vi "ECA200.vi"() -> ()   [LabVIEW 2020]
uses:
  <vilib>/Utility/miscctls.llb/LVComboBoxStrsAndValuesArrayTypeDef.ctl
panel:
  out "写入缓冲区":string
  in  "询问模式":bool
  out "返回数":u32
  out "读取缓冲区":string
  in  "测量":bool
  in  "确定按钮":bool
  in  "值":string(combo)
  in  "测量项":string(combo)
  in  "设置项":string(combo)
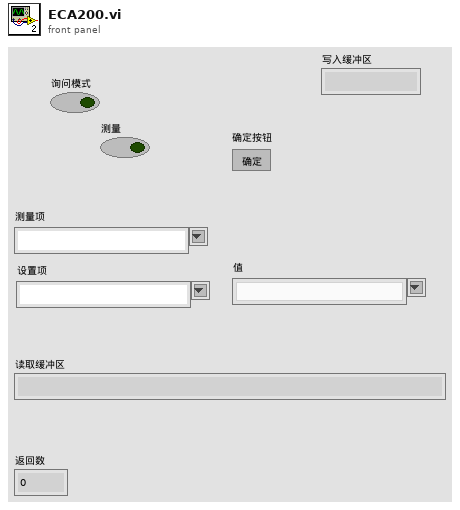
[diagram p1: front panel]
types:
  T1 = typedef "LVComboBoxStrsAndValuesArrayTypeDef.ctl" = cluster{"String":string, "Value":string}[]
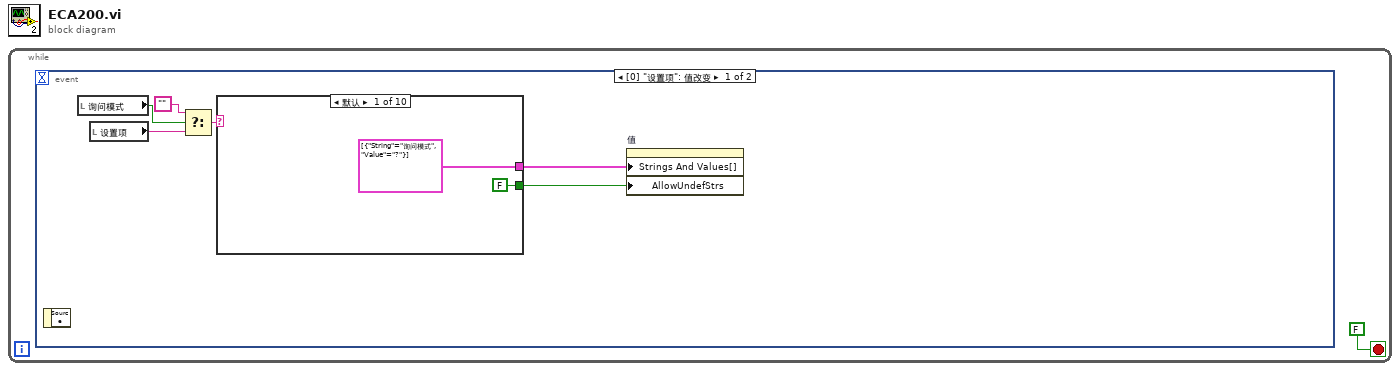
[diagram p0: block diagram]
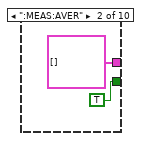
[diagram p2: hidden frame]
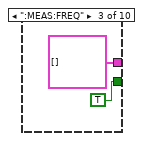
[diagram p3: hidden frame]
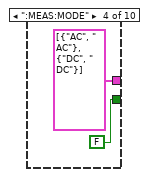
[diagram p4: hidden frame]
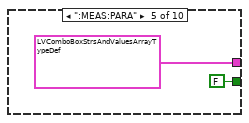
[diagram p5: hidden frame]
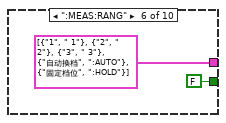
[diagram p6: hidden frame]
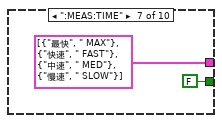
[diagram p7: hidden frame]
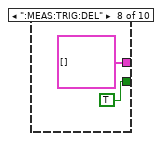
[diagram p8: hidden frame]
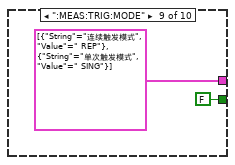
[diagram p9: hidden frame]
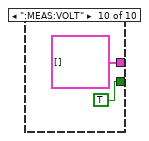
[diagram p10: hidden frame]
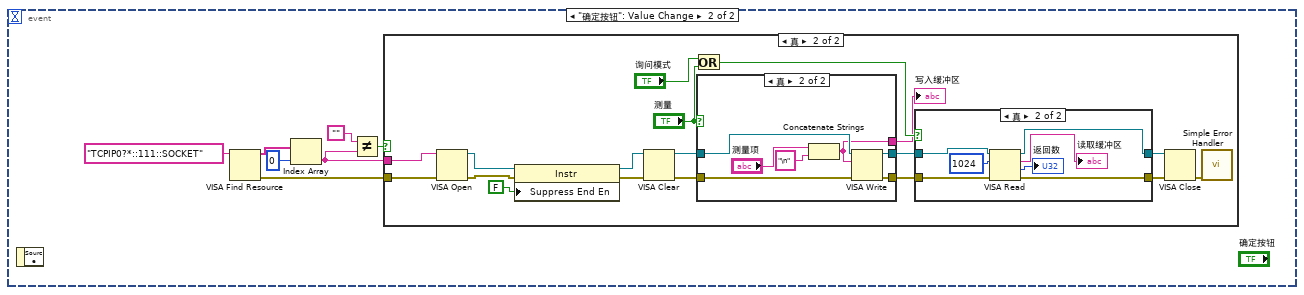
[diagram p11: hidden frame]
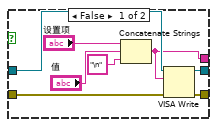
[diagram p14: hidden frame]
diagram:
  n1 = while {
    stop <- FALSE stop-if-true
    n2 = event shown="[0] \"设置项\": 值改变" {
      selector: _ -> [_ _]
      dyn-events: _ -> [_ _]
      timeout: _ -> [_ _]
      event "设置项": Value Change {
        n3 = event-data() -> ()  [unwired: 1 in, 1 out]
        n4 = local read "询问模式"() -> (w2:bool)
        n5 = local read "设置项"() -> (w5:string)
        n6 = Select(t="", s=w2, f=w5) -> (s? t:f=w7:string)
        n7 = case shown="默认" w7 {
          tunnel: [T1 [{"String"="询问模式", "Value"="?"}] ("字符串与值[]") T1 [] ("字符串与值[]") T1 [] ("字符串与值[]") T1 [{"String"="AC", "Value"=" AC"}, {"String"="DC", "Value"=" DC"}] ("字符串与值[]") T1 [{"String"="串联电感(Ls)", "Value"=" LS"}, {"String"="并联电感(Lp)", "Value"=" LP"}, {"String"="串联电容(Cs)", "Value"=" CS"}, {"String"="并联电容(Cp)", "Value"=" CP"}, {"String"="串联电阻(Rs)", "Value"=" RS"}, {"String"="并联电阻(Rp)", "Value"=" RP"}, {"String"="电抗(X)", "Value"=" X"}, {"String"="电纳(B)", "Value"=" B"}, {"String"="阻抗(Z)", "Value"=" Z"}, {"String"="导纳(Y)", "Value"=" Y"}, {"String"="损耗因数(D)", "Value"=" D"}, {"String"="品质因数(Q)", "Value"=" Q"}, {"String"="相位角(θ)", "Value"=" DEG"}, {"String"="电导(G)", "Value"=" G"}] ("字符串与值[]") T1 [{"String"="1", "Value"=" 1"}, {"String"="2", "Value"=" 2"}, {"String"="3", "Value"=" 3"}, {"String"="自动换档", "Value"=":AUTO"}, {"String"="固定档位", "Value"=":HOLD"}] ("字符串与值[]") T1 [{"String"="最快", "Value"=" MAX"}, {"String"="快速", "Value"=" FAST"}, {"String"="中速", "Value"=" MED"}, {"String"="慢速", "Value"=" SLOW"}] ("字符串与值[]") T1 [] ("字符串与值[]") T1 [{"String"="连续触发模式", "Value"=" REP"}, {"String"="单次触发模式", "Value"=" SING"}] ("字符串与值[]") T1 [] ("字符串与值[]")] -> w4
          tunnel: [FALSE TRUE TRUE FALSE FALSE FALSE FALSE TRUE FALSE TRUE] -> w3
          frame Default {
          }
          frame ":MEAS:AVER" {
          }
          frame ":MEAS:FREQ" {
          }
          frame ":MEAS:MODE" {
          }
          frame ":MEAS:PARA" {
          }
          frame ":MEAS:RANG" {
          }
          frame ":MEAS:TIME" {
          }
          frame ":MEAS:TRIG:DEL" {
          }
          frame ":MEAS:TRIG:MODE" {
          }
          frame ":MEAS:VOLT" {
          }
        }
        n8 = property on="值" class="CmbBox"("Strings And Values[]"=w4, "AllowUndefStrs"=w3) -> ()  [unwired: 2 in, 2 out]
      }
      event "确定按钮": Value Change {
        n9 = event-data() -> ()  [unwired: 1 in, 1 out]
        n10 = VISA Find Resource(11:"TCPIP0?*::111::SOCKET" ("表达式(\"?*\")")) -> (0:w32:errorcluster, 3:w31:string[])  [unwired: 2 in, 1 out]
        n11 = Index Array(array=w31, index=0 ("索引")) -> (element=w33:string)
        n12 = Not Equal?(x="", y=w33) -> (x != y?=w34:bool)
        n13 = case shown="真" w34 {
          tunnel: w32 -> [_ w44]
          tunnel: w33 -> [_ w43]
          frame False {
          }
          frame True {
            n14 = VISA Open(error in (no error)=w44, VISA resource name=w43) -> (VISA resource name=w46:refnum<visa-resource-name>, error out=w45:errorcluster)  [unwired: 3 in]
            n15 = property class="Instr"(reference=w46, error in=w45, "Suppress End En"=FALSE ("Message Based Settings:Suppress End Enable")) -> (reference out=w48:refnum<visa-resource-name>, error out=w47:errorcluster)
            n16 = VISA Clear(VISA resource name=w48, error in (no error)=w47) -> (VISA resource name out=w52:refnum<visa-resource-name>, error out=w51:errorcluster)
            n17 = Or(x="询问模式", y="测量") -> (x .or. y?=w38:bool)
            n18 = case shown="真" "测量" {
              tunnel: w52 -> [w69 w76]
              tunnel: w51 -> [w68 w75]
              tunnel: [w67 w72] -> w42
              tunnel: [w66 w71] -> w41
              tunnel: [w62 w70] -> w35
              frame False {
                n19 = Concatenate Strings("设置项", "值", "\n" ("字符串")) -> (w62:string)
                n20 = VISA Write(VISA resource name=w69, write buffer=w62, error in (no error)=w68) -> (VISA resource name out=w67:refnum<visa-resource-name>, error out=w66:errorcluster)  [unwired: 1 out]
              }
              frame True {
                n21 = Concatenate Strings("测量项", "\n" ("字符串")) -> (w70:string)
                n22 = VISA Write(VISA resource name=w76, write buffer=w70, error in (no error)=w75) -> (VISA resource name out=w72:refnum<visa-resource-name>, error out=w71:errorcluster)  [unwired: 1 out]
              }
            }
            "写入缓冲区" <- w35
            n23 = case shown="真" w38 {
              tunnel: w42 -> [w54 w58]
              tunnel: w41 -> [w53 w57]
              tunnel: [w53 w56] -> w40
              tunnel: [w54 w55] -> w39
              frame False {
              }
              frame True {
                n24 = VISA Read(VISA resource name=w58, byte count=u32 1024 ("字节总数"), error in (no error)=w57) -> (VISA resource name out=w55:refnum<visa-resource-name>, read buffer=→"读取缓冲区":string, return count=→"返回数":u32, error out=w56:errorcluster)
              }
            }
            n25 = VISA Close(VISA resource name=w39, error in (no error)=w40) -> (error out=w49:errorcluster)
            n26 = call <vilib>:"Simple Error Handler.vi"("error in (no error)"=w49) -> ()  [unwired: 4 in, 5 out]
          }
        }
      }
    }
  }
